vi "Configure IR Range Upper.vi"(8 "error in (no error)":errorcluster, 9 "Value":dbl min=0.0 max=0.01 format="%.2p", 10 "Step":T1=1 min=1 max=99 step=1, 11 "VISA resource name":refnum<visa-resource-name>) -> (0 "error out":errorcluster, 3 "VISA resource name out":refnum<visa-resource-name>)   [LabVIEW 2025, in "Chroma 19052.lvlib"]
uses:
  <instrlib>/Chroma 19052/Chroma 19052.lvlib
  <instrlib>/Chroma 19052/Public/Utility/Type Def/steps--numeric.ctl
panel:
  # "Configure RANGE UPPER"
  # "(for IR mode ONLY)"
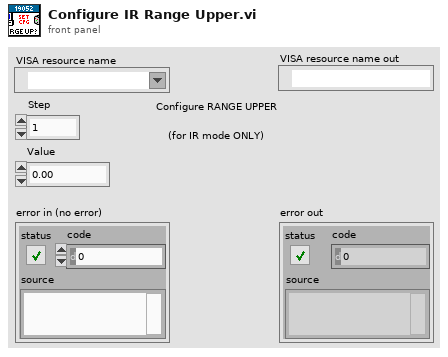
[diagram p1: front panel]
types:
  T1 = typedef "Chroma 19052.lvlib/steps--numeric.ctl" = u8
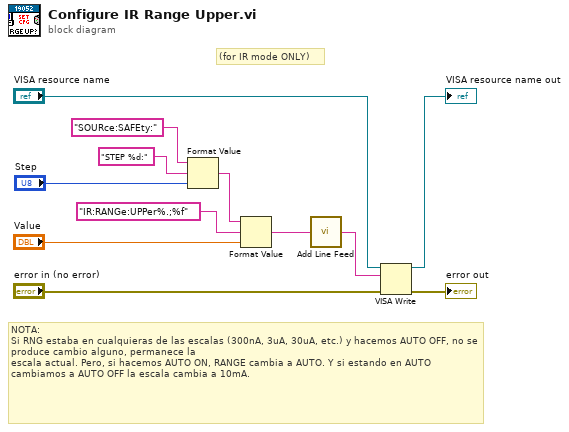
[diagram p0: block diagram]
diagram:
  # "(for IR mode ONLY)"
  # "NOTA: \nSi RNG estaba en cualquieras de las escalas (300nA, 3uA, 30uA, etc.) y hacemos AUTO OFF, no se produce cambio alguno, permanece la\nescala actual. Pero, si hacemos AUTO ON, RANGE cambia a AUTO. Y si estando en AUTO cambiamos a AUTO OFF la escala cambia a 10mA."
  n1 = Format Value(string ("")="SOURce:SAFEty:", format string="STEP %d:", value (0)="Step") -> (output string=w4:string)
  n2 = Format Value(string ("")=w4, format string="IR:RANGe:UPPer%.;%f", value (0)="Value") -> (output string=w3:string)
  n3 = call <instrlib>:"Add Line Feed.vi"("Command string"=w3) -> ("Concatenated string"=w8:string)  [unwired: 4 in]
  n4 = VISA Write(VISA resource name="VISA resource name", write buffer=w8, error in (no error)="error in (no error)") -> (VISA resource name out=→"VISA resource name out":refnum<visa-resource-name>, error out=→"error out":errorcluster)  [unwired: 1 out]
